vi "Log RTD.vi"(8 "error in 2":errorcluster, 10 "Queue Ref":T1, 11 "tdms file in 2":refnum<k34>) -> (0 "error out 2":errorcluster, 3 "tdms file in":refnum<k34>)   [LabVIEW 2022 SP3]
uses:
  Controls/All Queue Ref.ctl
  <vilib>/Waveform/WDTOps.llb/WDT Get Waveform Time Array DBL.vi
panel:
  out "x":u32
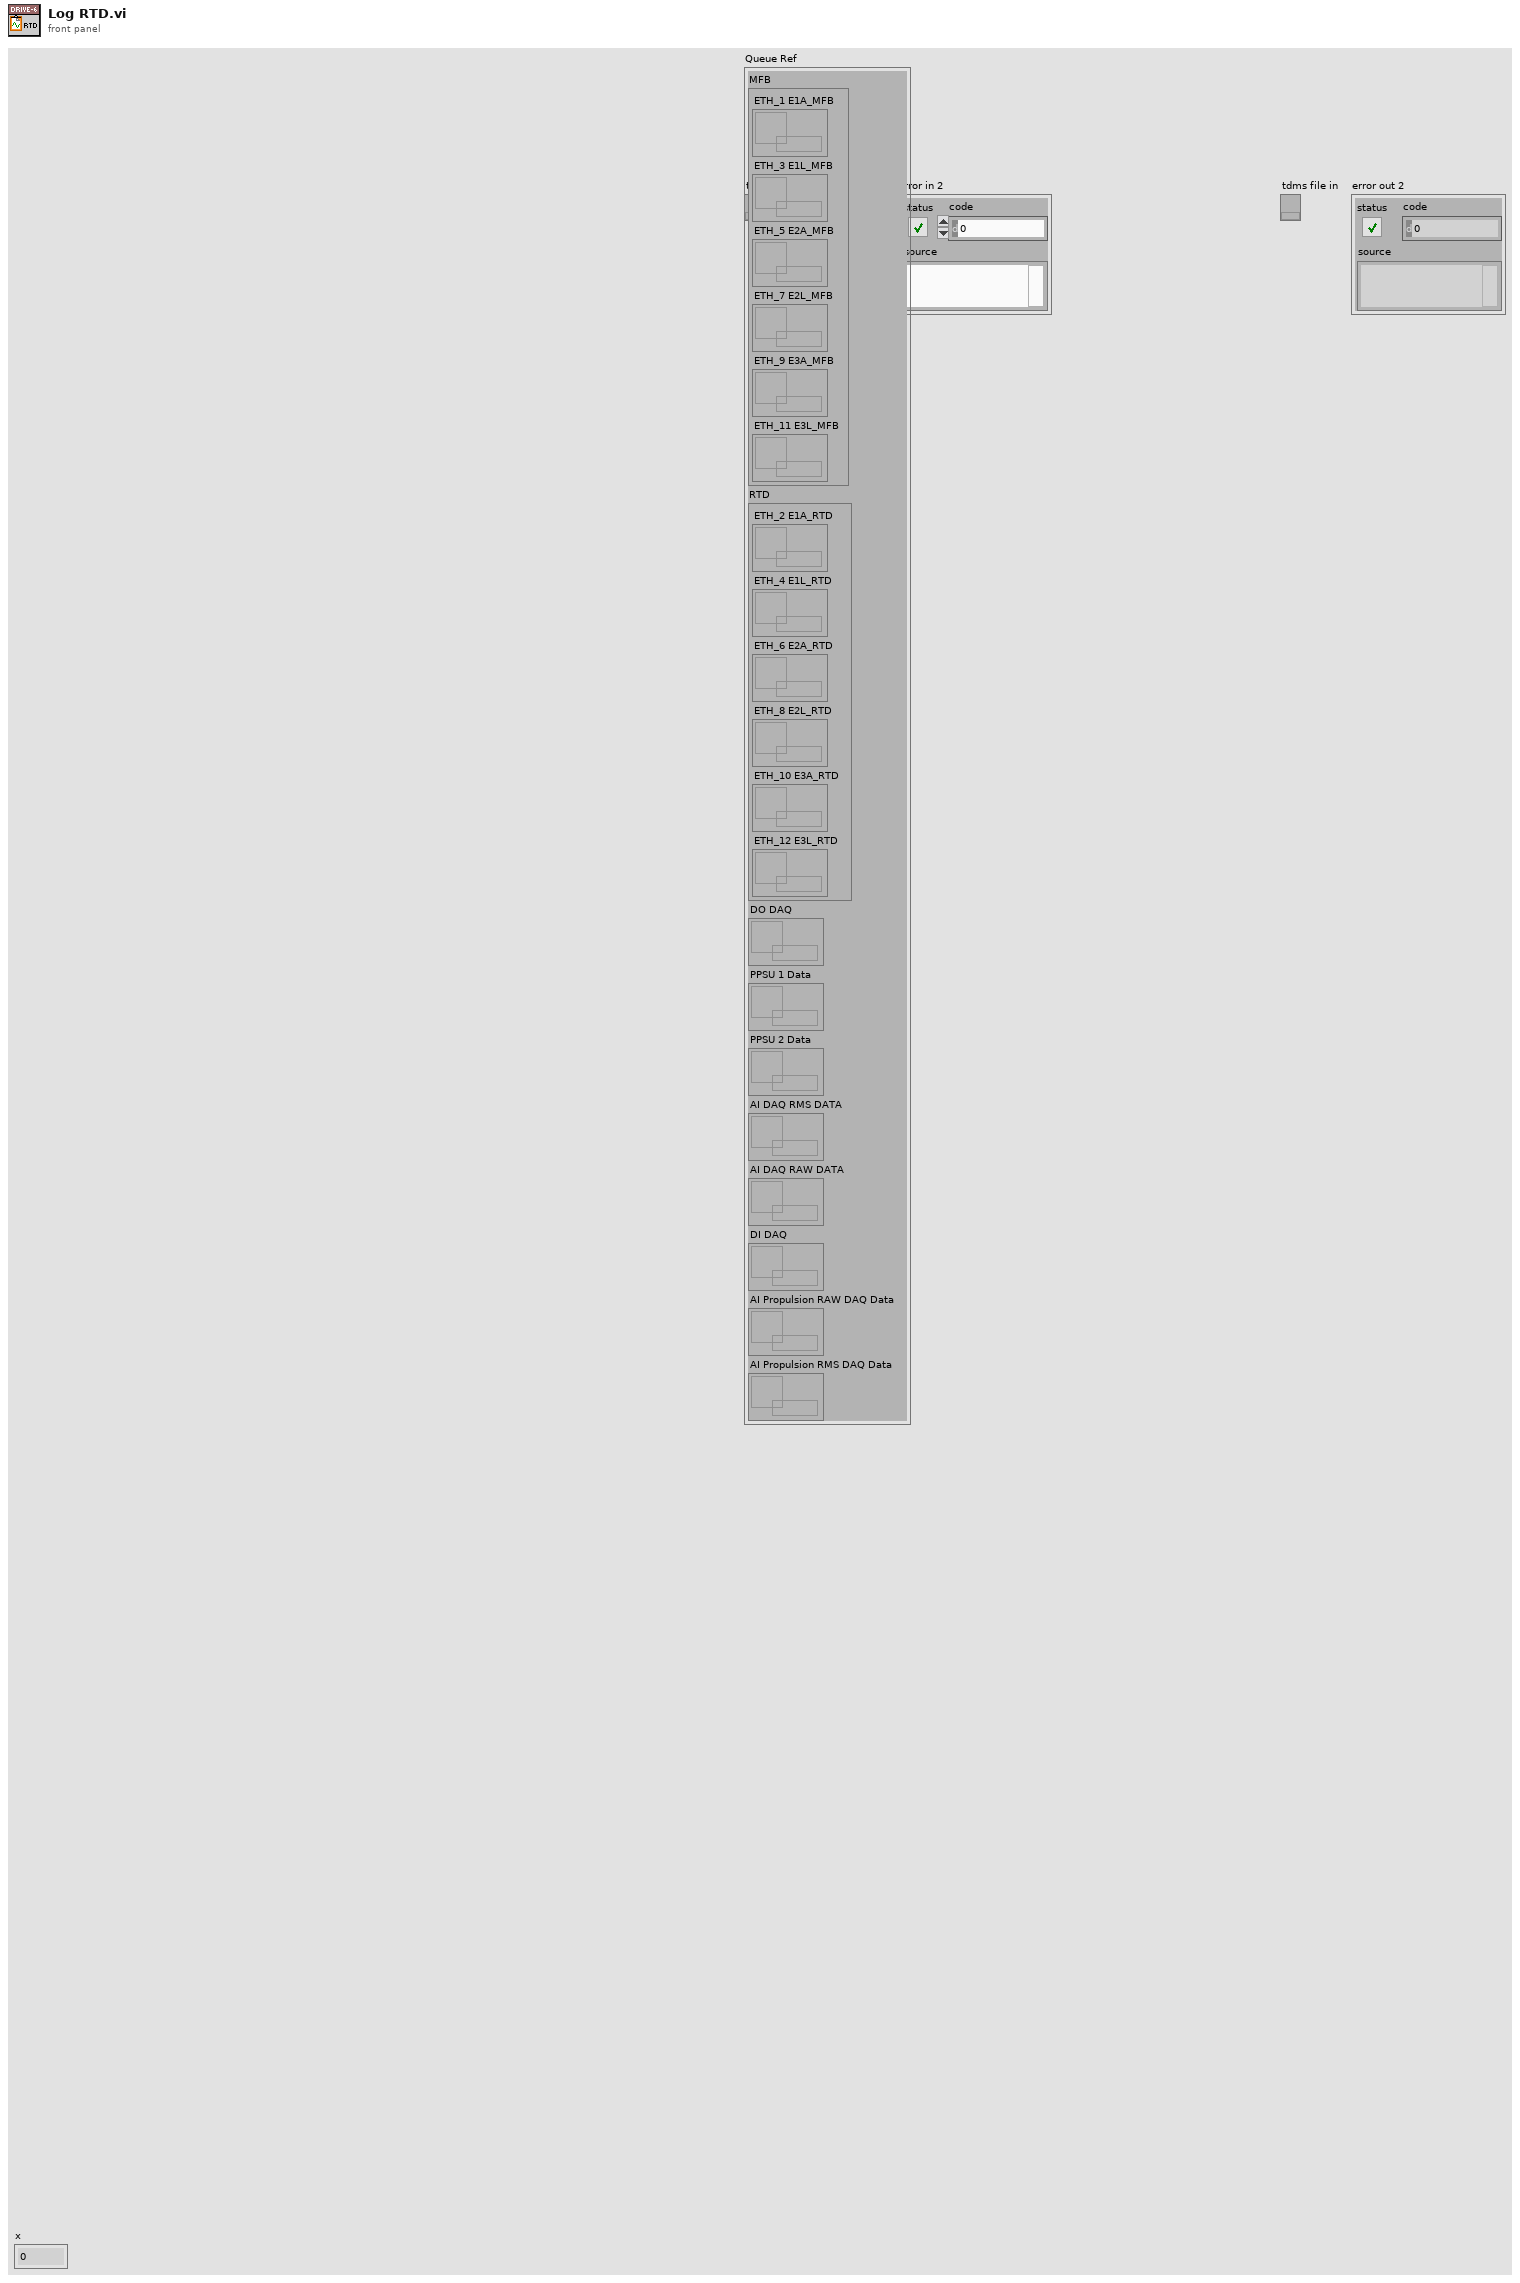
[diagram p1: front panel]
types:
  T1 = typedef "All Queue Ref.ctl" = cluster{"MFB":cluster{"ETH_1 E1A_MFB":refnum<queue>, "ETH_3 E1L_MFB":refnum<queue>, "ETH_5 E2A_MFB":refnum<queue>, "ETH_7 E2L_MFB":refnum<queue>, "ETH_9 E3A_MFB":refnum<queue>, "ETH_11 E3L_MFB":refnum<queue>}, "RTD":cluster{"ETH_2 E1A_RTD ":refnum<queue>, "ETH_4 E1L_RTD ":refnum<queue>, "ETH_6 E2A_RTD ":refnum<queue>, "ETH_8 E2L_RTD ":refnum<queue>, "ETH_10 E3A_RTD ":refnum<queue>, "ETH_12 E3L_RTD ":refnum<queue>}, "DO DAQ":refnum<queue>, "PPSU 1 Data":refnum<queue>, "PPSU 2 Data":refnum<queue>, "AI DAQ RMS DATA":refnum<queue>, "AI DAQ RAW DATA":refnum<queue>, "DI DAQ":refnum<queue>, "AI Propulsion RAW DAQ Data":refnum<queue>, "AI Propulsion RMS DAQ Data":refnum<queue>}
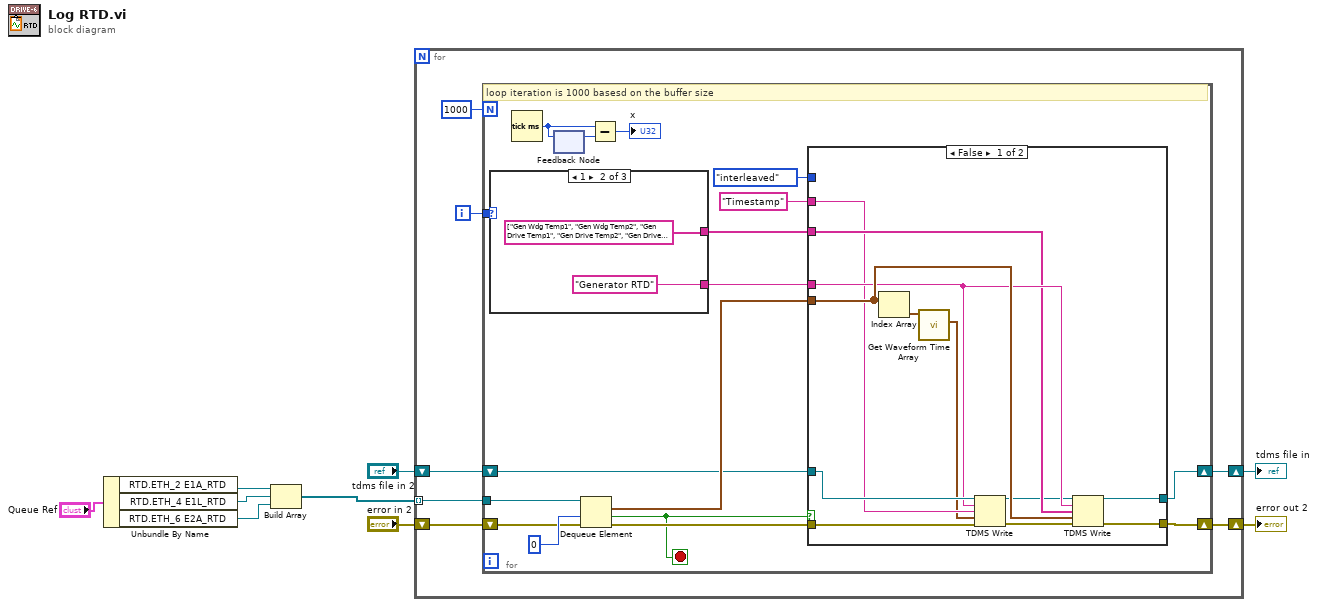
[diagram p0: block diagram]
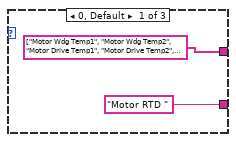
[diagram p3: hidden frame]
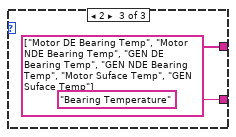
[diagram p4: hidden frame]
diagram:
  n1 = Unbundle By Name("Queue Ref") -> ("RTD.ETH_2 E1A_RTD"=w5:refnum<queue>, "RTD.ETH_4 E1L_RTD"=w4:refnum<queue>, "RTD.ETH_6 E2A_RTD"=w1:refnum<queue>)
  n2 = Build Array(w5, w4, w1) -> (w3:refnum<queue>[])
  n3 = for {
    tunnel: w3 -> [w15] mode=indexing
    shift-right: [w13] -> w7
    shift-left: "tdms file in 2" -> [w16]
    shift-right: [w11] -> w6
    shift-left: "error in 2" -> [w12]
    i -> [w10]
    n4 = for {
      N: 1000 -> [_]
      tunnel: w15 -> [w31]
      shift-right: [w23] -> w13
      shift-left: w16 -> [w21]
      shift-right: [w22] -> w11
      shift-left: w12 -> [w30]
      tunnel: w10 -> [w33]
      stop <- w19 stop-if-true
      # "loop iteration is 1000 basesd on the buffer size"
      n5 = case shown="1" w33 {
        tunnel: [string[] ["Motor Wdg Temp1", "Motor Wdg Temp2", "Motor Drive Temp1", "Motor Drive Temp2", "Motor Drive Temp3", "Motor Drive Temp4"] ("appended array") string[] ["Gen Wdg Temp1", "Gen Wdg Temp2", "Gen Drive Temp1", "Gen Drive Temp2", "Gen Drive Temp3", "Gen Drive Temp4"] ("appended array") string[] ["Motor DE Bearing Temp", "Motor NDE Bearing Temp", "GEN DE Bearing Temp", "GEN NDE Bearing Temp", "Motor Suface Temp", "GEN Suface Temp"] ("appended array")] -> w24
        tunnel: ["Motor RTD " ("group name in (Untitled)") "Generator RTD" ("group name in (Untitled)") "Bearing Temperature" ("group name in (Untitled)")] -> w25
        frame 0, Default {
        }
        frame 1 {
        }
        frame 2 {
        }
      }
      n6 = Tick Count (ms)() -> (millisecond timer value=w28:u32)
      n7 = feedback #1() -> (w29:u32)  [unwired: 1 in]
      n8 = feedback-in #1(w28) -> ()
      n9 = Dequeue Element(queue=w31, timeout in ms (-1)=0, error in (no error)=w30) -> (element=w26:waveform(dbl)[], timed out?=w19:bool, error out=w20:errorcluster)  [unwired: 1 out]
      n10 = Subtract(x=w28, y=w29) -> (x-y=→"x":u32)
      n11 = case shown="False" w19 {
        tunnel: [w45 w46] -> w22
        tunnel: [w44 w47] -> w23
        tunnel: w25 -> [w40 _]
        tunnel: "Timestamp" -> [w38 _]
        tunnel: w24 -> [w39 _]
        tunnel: w26 -> [w41 _]
        tunnel: enum16{"decimated", "interleaved"}."interleaved" ("data layout (0:decimated)") -> [_ _]
        tunnel: w21 -> [w42 w47]
        tunnel: w20 -> [w43 w46]
        frame False {
          n12 = Index Array(array=w41) -> (element=w35:waveform(dbl))  [unwired: 1 in]
          n13 = call-poly <vilib>:"Get Waveform Time Array.vi"("waveform in"=w35) -> ("X array"=w34:timestamp[])  [unwired: 9 in, 1 out]
          n14 = TDMS Write(0:w42, 5:w40, 7:w38, 9:w34, 11:w43) -> (4:w36:refnum<k34>, 15:w37:errorcluster)  [unwired: 1 in, 2 out]
          n15 = TDMS Write(0:w36, 5:w40, 7:w39, 9:w41, 11:w37) -> (4:w44:refnum<k34>, 15:w45:errorcluster)  [unwired: 1 in, 2 out]
        }
        frame True {
        }
      }
    }
  }
  "tdms file in" <- w7
  "error out 2" <- w6
